vi "GetText.vi"(8 "error in (no error)":errorcluster, 11 "3D Object in":refnum<class "3D Object.lvclass">) -> (0 "error out":errorcluster, 1 "Font Path":path, 2 "Text":string, 3 "3D Object out":refnum<class "3D Object.lvclass">, 4 "Alignment":T1, 5 "Alpha":sgl, 7 "Color":u32(colorbox))   [LabVIEW 2015, in "3D Object.lvclass"]
uses:
  3D Object.lvclass
  <vilib>/Utility/miscctls.llb/LVSceneTextAlignment.ctl
  3D Object.lvclass/3D Object.ctl
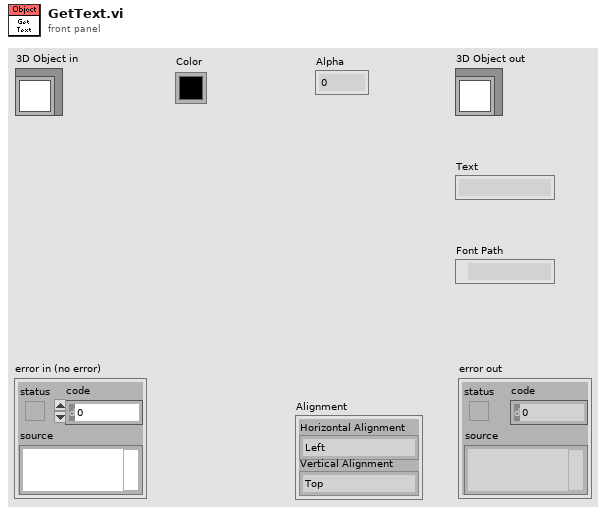
[diagram p1: front panel]
types:
  T1 = typedef "LVSceneTextAlignment.ctl" = cluster{"Horizontal Alignment":enum8{"Left", "Right", "Center"}, "Vertical Alignment":enum8{"Top", "Bottom", "Center", "Base Line", "Bottom Base Line"}}
  T2 = typedef "LVRGBAColorTypeDef.ctl" = cluster{"Red":sgl, "Green":sgl, "Blue":sgl, "Alpha":sgl}
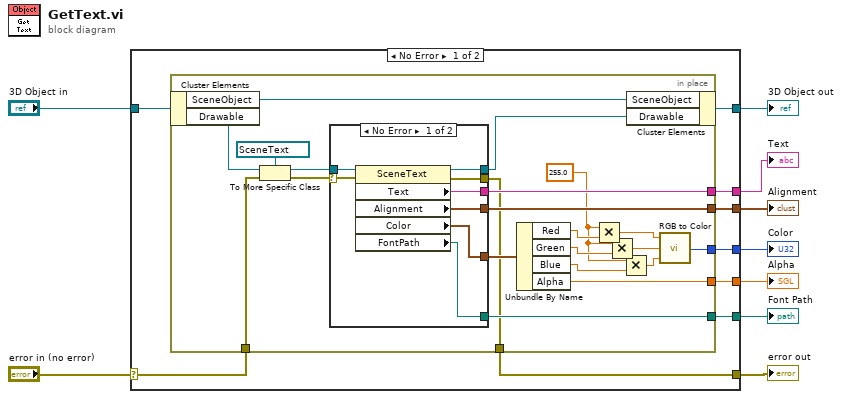
[diagram p0: block diagram]
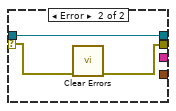
[diagram p2: hidden frame]
diagram:
  n1 = case shown="No Error" "error in (no error)" {
    selector: "error in (no error)" -> [w17 w52]
    tunnel: [w16 w52] -> w8
    tunnel: [w10 w51] -> w6
    tunnel: "3D Object in" -> [w18 w51]
    tunnel: [w15 _] -> w5
    tunnel: [w14 _] -> w4
    tunnel: [w13 _] -> w3
    tunnel: [w12 _] -> w2
    tunnel: [w11 _] -> w1
    frame No Error {
      n2 = in-place {
        in-place-border: w17 -> [w28]
        in-place-border: [w26] -> w16
        in-place-border: [w36] -> w15
        in-place-border: [w35] -> w14
        in-place-border: [w34] -> w13
        in-place-border: [w32] -> w12
        in-place-border: [w31] -> w11
        w20 = sgl 255.0 ("x")
        n3 = in-place-cluster #1(w18) -> ("SceneObject"=w30:refnum<vi>, "Drawable"=w29:refnum<vi>)
        n4 = To More Specific Class(target class=refnum<vi> refnum ("reference"), reference=w29, error in=w28) -> (specific class reference=w38:refnum<vi>, error out=w37:errorcluster)
        n5 = case shown="No Error" w37 {
          selector: w37 -> [w46 w50]
          tunnel: w38 -> [w47 w48]
          tunnel: [w45 w48] -> w27
          tunnel: [w44 w49] -> w26
          tunnel: [w43 _] -> w36
          tunnel: [w42 _] -> w35
          tunnel: [w41 _] -> w33
          tunnel: [w40 _] -> w34
          frame No Error {
            n6 = property class="SceneText"(reference=w47, error in=w46) -> (reference out=w45:refnum<vi>, error out=w44:errorcluster, "Text"=w43:string, "Alignment"=w42:T1, "Color"=w41:T2, "FontPath"=w40:path)
          }
          frame Error {
            n7 = call <vilib>:"Clear Errors.vi"("error in (no error)"=w50) -> ("error out"=w49:errorcluster)  [unwired: 5 in, 1 out]
          }
        }
        n8 = Unbundle By Name(w33) -> ("Red"=w25:sgl, "Green"=w24:sgl, "Blue"=w21:sgl, "Alpha"=w31:sgl)
        n9 = Multiply(x=w20, y=w25) -> (x*y=w22:sgl)
        n10 = Multiply(x=w20, y=w24) -> (x*y=w23:sgl)
        n11 = Multiply(x=w20, y=w21) -> (x*y=w19:sgl)
        n12 = in-place-cluster #1("SceneObject"=w30, "Drawable"=w27) -> (w10:refnum<class "3D Object.lvclass">)
        n13 = call <vilib>:"RGB to Color.vi"("B"=w19, "G"=w23, "R"=w22) -> ("Color"=w32:u32)
      }
    }
    frame Error {
    }
  }
  "error out" <- w8
  "3D Object out" <- w6
  "Text" <- w5
  "Alignment" <- w4
  "Font Path" <- w3
  "Color" <- w2
  "Alpha" <- w1
